vi "File Directory Path Count.vi"(8 "error in (no error)":errorcluster, 9 "Directory (\"D:\\user\\data\")":string="D:\\user\\data", 10 "Read (Subdirectories and Files)":i32(ring) items=["Subdirectories and Files", "Subdirectories"], 11 "VISA resource name":refnum<visa-resource-name>) -> (0 "error out":errorcluster, 2 "Numbers of dir":i32, 3 "VISA resource name out":refnum<visa-resource-name>)   [LabVIEW 2020, in "Rohde&Schwarz CMXP Base.lvlib"]
doc: "This VI returns the number of files and/or subdirectories of the current or of a specified directory. The number includes the parent directory strings \".\" and \"..\" so that it corresponds to the number of strings returned by the File Directory Path VI after the initial numeric parameters.\n\nAttribute:\n-\n\nRemote-control commands:\nMMEMory:CATalog:LENGth?\nMMEMory:DCATalog:LENGth?"
uses:
  <instrlib>/Rohde&Schwarz CMXP Base/Rohde&Schwarz CMXP Base.lvlib
  <instrlib>/Rohde&Schwarz CMXP Base/Private/rsidr_core.llb/rsidr_core.lvlib
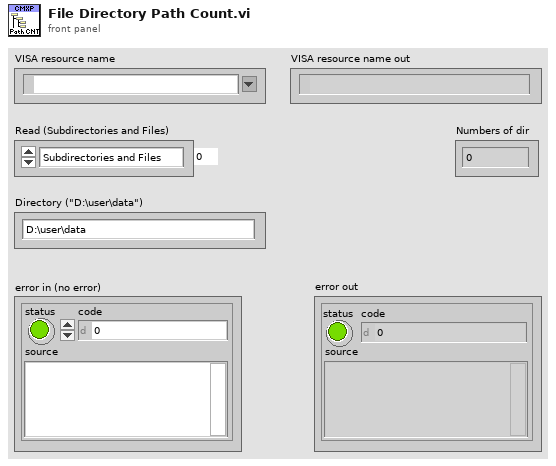
[diagram p1: front panel]
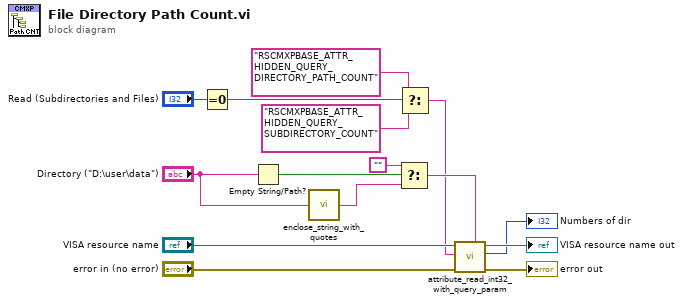
[diagram p0: block diagram]
diagram:
  n1 = Equal To 0?(x="Read (Subdirectories and Files)") -> (x = 0?=w10:bool)
  n2 = Empty String/Path?(string/path="Directory (\"D:\\user\\data\")") -> (empty?=w9:bool)
  n3 = call <instrlib>:"enclose_string_with_quotes.vi"("String to enclose"="Directory (\"D:\\user\\data\")") -> ("String out"=w1:string)  [unwired: 4 in]
  n4 = Select(t="" ("Empty String Constant"), s=w9, f=w1) -> (s? t:f=w7:string)
  n5 = Select(t="RSCMXPBASE_ATTR_HIDDEN_QUERY_DIRECTORY_PATH_COUNT", s=w10, f="RSCMXPBASE_ATTR_HIDDEN_QUERY_SUBDIRECTORY_COUNT") -> (s? t:f=w6:string)
  n6 = call <instrlib>:"attribute_read_int32_with_query_param.vi"("Query Parameter (None)"=w7, "error in"="error in (no error)", "Attribute ID"=w6, "VISA resource name"="VISA resource name") -> ("error out"=→"error out":errorcluster, "Int32 out"=→"Numbers of dir":i32, "VISA resource name out"=→"VISA resource name out":refnum<visa-resource-name>)  [unwired: 5 in]
